vi "Calibrate_Open_All_Freqs-NEW.vi"(8 "error in":errorcluster, 10 "Stop Test":bool, 11 "Calibration Test":bool) -> (0 "error out":errorcluster, 5 "Open Calibration Successful":bool)   [LabVIEW 2020]
uses:
  <vilib>/Utility/error.llb/DialogType.ctl
panel:
  out "message":string=" INSTRUCTIONS:\r\rNormal Use:  When using subVIs that incorporate the error in/error out (or error I/O) structure, place this handler where you want to inform the user of an error, typically at the end of the I/O data path, as the last action of the program.  If the error in error? is ERROR, the handler creates a message describing the error and its source.  If the type of dialog = 1 (default), the message is displayed to the user, who can only acknowedge it.  If the type = 2, the user can acknowledge the message or abort execution; aborting a program with active I/O is not recommended.  If the type = 0, no message is displayed; this is used to process the error programmatically, and the error out cluster elements are wired to individual terminals for that reason.  \r\rOther Use:\n\r\nlocal testing.  To test the error code of a subVI or function that does not have the error I/O structure, you can wire its error code and a source string to the local error code and error source inputs.  If error in error? indicates no error and error code is not equal to 0, the local code and source are substituted for the error in values, and error? is set TRUE (ERROR)."
  out "Test Count":i32
  out "Failed Test Count":i32
  in  "Cal_Delay_Step":u16
  out "serial poll byte":i16
  in  "Test Failed":bool
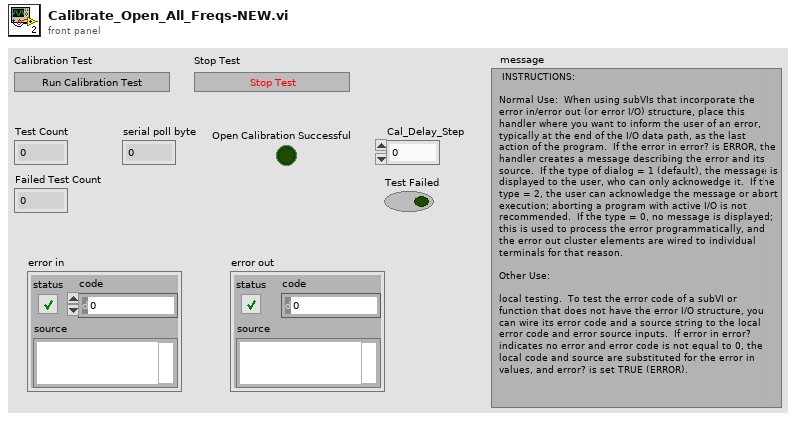
[diagram p1: front panel]
types:
  T1 = typedef "DialogType.ctl" = u16
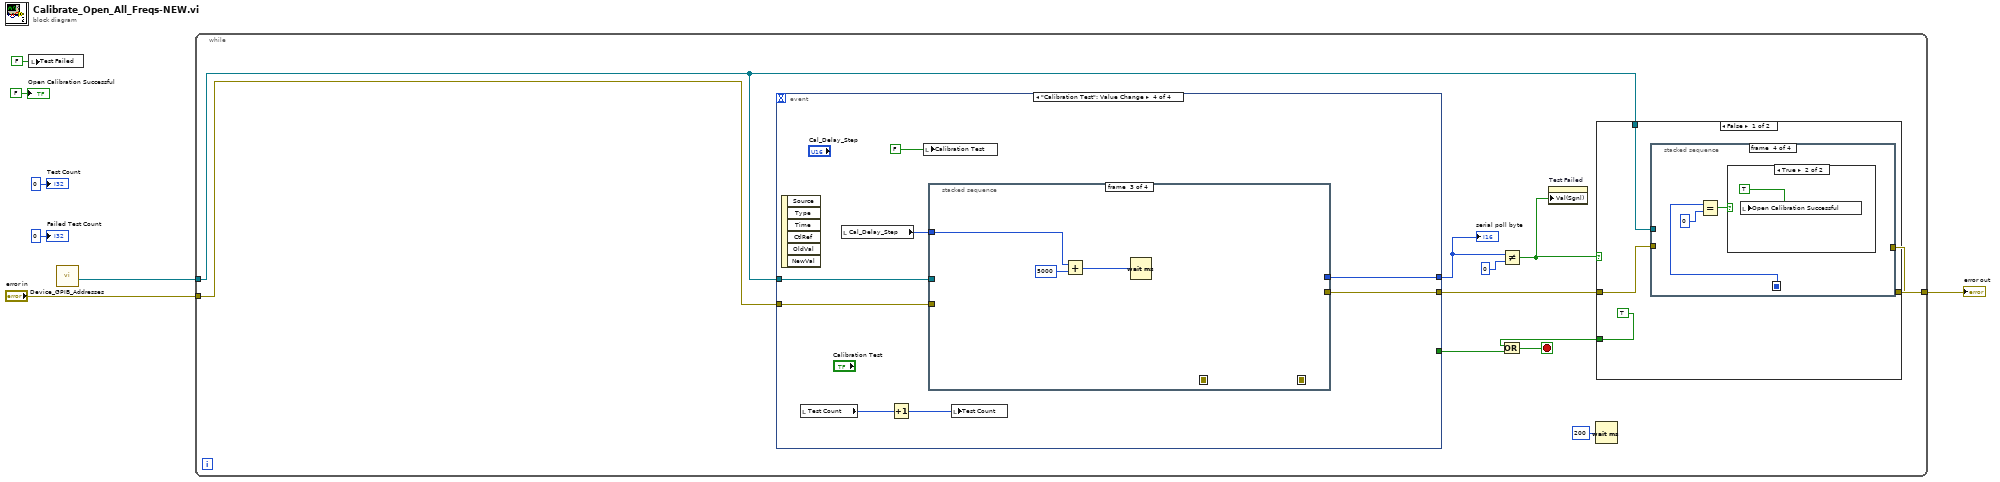
[diagram p0: block diagram]
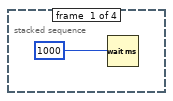
[diagram p2: hidden frame]
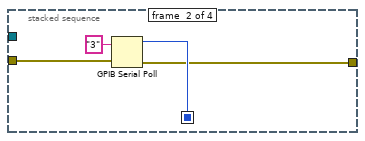
[diagram p3: hidden frame]
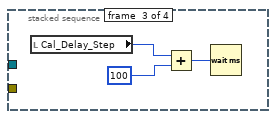
[diagram p4: hidden frame]
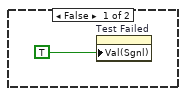
[diagram p5: hidden frame]
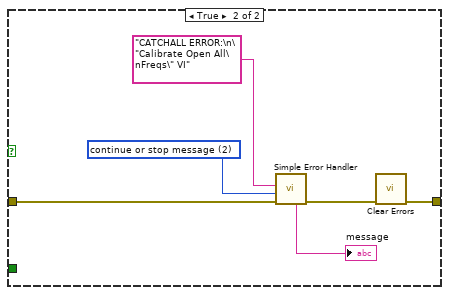
[diagram p6: hidden frame]
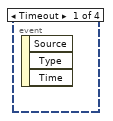
[diagram p7: hidden frame]
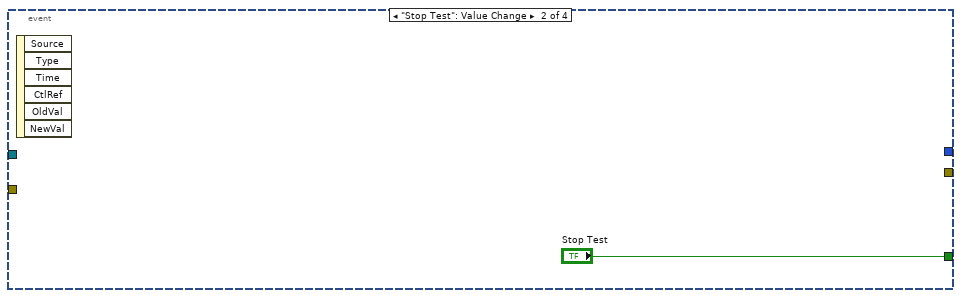
[diagram p8: hidden frame]
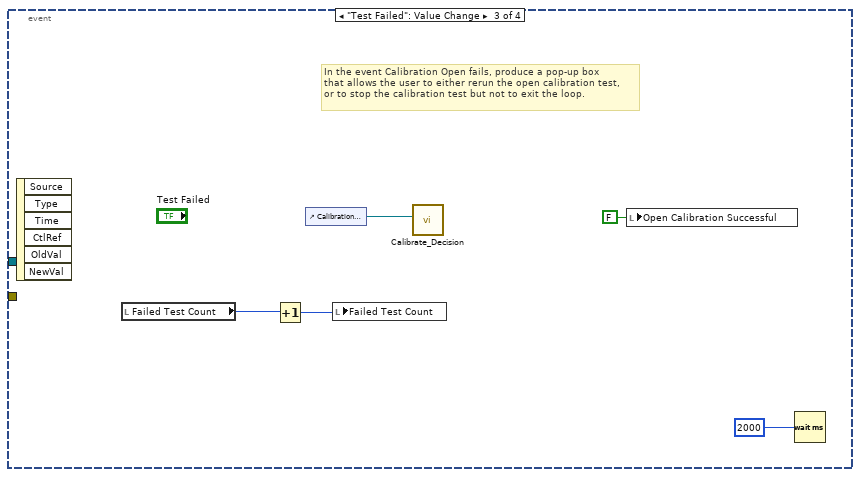
[diagram p9: hidden frame]
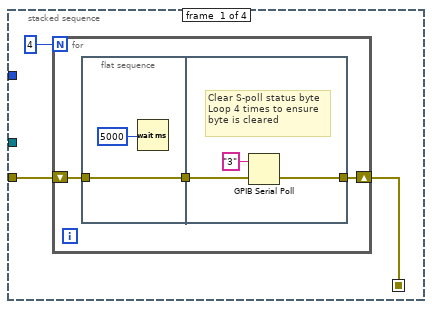
[diagram p10: hidden frame]
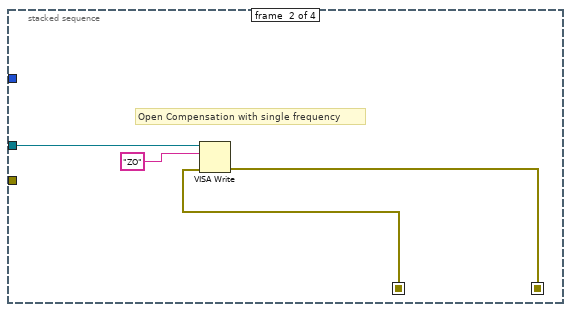
[diagram p11: hidden frame]
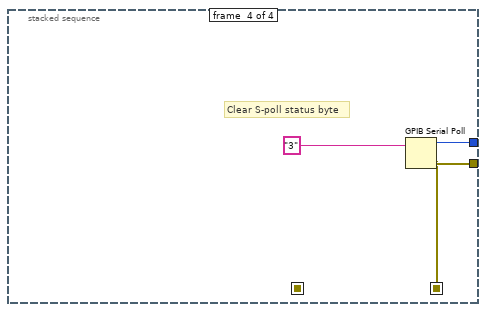
[diagram p12: hidden frame]
diagram:
  n1 = local write "Test Failed"(FALSE ("Test Failed")) -> ()
  n2 = call "Device_GPIB_Addresses.vi"() -> ("HP 4275A Address"=w5:refnum<visa-resource-name>)  [unwired: 9 in, 2 out]
  n3 = while {
    tunnel: w5 -> [w9]
    tunnel: [w17] -> w4
    tunnel: "error in" -> [w8]
    stop <- w13 stop-if-true
    n4 = event shown="[3] \"Calibration Test\": Value Change" {
      selector: _ -> [_ _ _ _]
      dyn-events: _ -> [_ _ _ _]
      timeout: _ -> [_ _ _ _]
      tunnel: [_ "Stop Test" _ _] -> w14
      tunnel: w9 -> [_ _ _ w51]
      tunnel: [_ _ _ w50] -> w18
      tunnel: [_ _ _ w49] -> w15
      tunnel: w8 -> [_ _ _ w48]
      event Timeout {
        n5 = event-data() -> ()  [unwired: 1 in, 3 out]
      }
      event "Stop Test": Value Change {
        n6 = event-data() -> ()  [unwired: 1 in, 6 out]
      }
      event "Test Failed": Value Change {
        # "In the event Calibration Open fails, produce a pop-up box\nthat allows the user to either rerun the open calibration test,\nor to stop the calibration test but not to exit the loop."
        n7 = event-data() -> ()  [unwired: 1 in, 6 out]
        n8 = local read "Failed Test Count"() -> (w45:i32)
        n9 = Increment(x=w45) -> (x+1=w46:i32)
        n10 = control-ref of="Calibration Test"() -> (w47:refnum<vi>)
        n11 = local write "Failed Test Count"(w46) -> ()
        n12 = call "Calibrate_Decision.vi"("reference"=w47) -> ()  [unwired: 11 in]
        n13 = local write "Open Calibration Successful"(FALSE ("Open Calibration Successful")) -> ()
        n14 = Wait (ms)(milliseconds to wait=u32 2000) -> ()  [unwired: 1 out]
      }
      event "Calibration Test": Value Change {
        n15 = event-data() -> ()  [unwired: 1 in, 6 out]
        n16 = local read "Test Count"() -> (w54:i32)
        n17 = local read "Cal_Delay_Step"() -> (w52:u16)
        n18 = Increment(x=w54) -> (x+1=w53:i32)
        n19 = local write "Calibration Test"(FALSE ("Calibration Test")) -> ()
        n20 = stacked-sequence {
          seq-local: [w56 _ _ _] -> [_ w68 _ _]
          seq-local: [_ w67 _ _] -> [_ _ _ w74]
          tunnel: w48 -> [w57 _ _ _]
          tunnel: w52 -> [_ _ w73 _]
          tunnel: [_ _ _ w77] -> w50
          tunnel: [_ _ _ w76] -> w49
          tunnel: w51 -> [_ w70 _ _]
          frame #0 {
            n21 = for {
              N: 4 -> [_]
              shift-right: [w60] -> w56
              shift-left: w57 -> [w61]
              n22 = flat-sequence {
                tunnel: w61 -> [w63]
                tunnel: [w63] -> w59
                tunnel: [w65] -> w60
                tunnel: w59 -> [w66]
                frame #0 {
                  n23 = Wait (ms)(milliseconds to wait=u32 5000) -> ()  [unwired: 1 out]
                }
                frame #1 {
                  # "Clear S-poll status byte\nLoop 4 times to ensure\nbyte is cleared"
                  n24 = GPIB Serial Poll(0:"3" ("address string"), 1:w66) -> (4:w65:errorcluster)  [unwired: 2 out]
                }
              }
            }
          }
          frame #1 {
            # "Open Compensation with single frequency"
            n25 = VISA Write(VISA resource name=w70, write buffer="ZO" ("data"), error in (no error)=w68) -> (error out=w67:errorcluster)  [unwired: 2 out]
          }
          frame #2 {
            n26 = Add(x=w73, y=u16 5000) -> (x+y=w71:u16)
            n27 = Wait (ms)(milliseconds to wait=w71) -> ()  [unwired: 1 out]
          }
          frame #3 {
            # "Clear S-poll status byte"
            n28 = GPIB Serial Poll(0:"3" ("address string"), 1:w74) -> (2:w76:i16, 4:w77:errorcluster)  [unwired: 1 out]
          }
        }
        n29 = local write "Test Count"(w53) -> ()
      }
    }
    "serial poll byte" <- w15
    n30 = Not Equal?(x=w15, y=i16 0) -> (x != y?=w11:bool)
    n31 = property on="Test Failed" class="Bool (strict)"("Val(Sgnl)"=w11) -> ()  [unwired: 2 in, 2 out]
    n32 = Wait (ms)(milliseconds to wait=u32 200) -> ()  [unwired: 1 out]
    n33 = case shown="False" w11 {
      tunnel: w9 -> [w22 _]
      tunnel: w18 -> [w21 w36]
      tunnel: [w20 w37] -> w17
      tunnel: [TRUE _] -> w12
      frame False {
        n34 = stacked-sequence {
          seq-local: [_ w25 _ _] -> [_ _ _ w33]
          tunnel: w21 -> [_ w27 _ _]
          tunnel: [_ w24 _ _] -> w20
          tunnel: w22 -> [_ _ _ _]
          frame #0 {
            n35 = Wait (ms)(milliseconds to wait=u16 1000 ("y")) -> ()  [unwired: 1 out]
          }
          frame #1 {
            n36 = GPIB Serial Poll(0:"3" ("address string"), 1:w27) -> (2:w25:i16, 4:w24:errorcluster)  [unwired: 1 out]
          }
          frame #2 {
            n37 = local read "Cal_Delay_Step"() -> (w28:u16)
            n38 = Add(x=w28, y=u16 100) -> (x+y=w29:u16)
            n39 = Wait (ms)(milliseconds to wait=w29) -> ()  [unwired: 1 out]
          }
          frame #3 {
            n40 = Equal?(x=w33, y=i16 0) -> (x = y?=w31:bool)
            n41 = case shown="True" w31 {
              frame False {
                n42 = property on="Test Failed" class="Bool (strict)"("Val(Sgnl)"=TRUE ("Test Failed")) -> ()  [unwired: 2 in, 2 out]
              }
              frame True {
                n43 = local write "Open Calibration Successful"(TRUE ("Open Calibration Successful")) -> ()
              }
            }
          }
        }
      }
      frame True {
        w39 = T1 2 items=["no dialog", "OK message", "continue or stop message", "OK message + warnings", "continue/stop + warnings"] ("type of dialog (OK msg:1)")
        n44 = call <vilib>:"Simple Error Handler.vi"("error source (\" \")"="CATCHALL ERROR:\n\"Calibrate Open All\nFreqs\" VI" ("error source (\" \")"), "type of dialog (OK msg:1)"=w39, "error in (no error)"=w36) -> ("error out"=w40:errorcluster, "message"=→"message":string)  [unwired: 2 in, 3 out]
        n45 = call <vilib>:"Clear Errors.vi"("error in (no error)"=w40) -> ("error out"=w37:errorcluster)  [unwired: 5 in, 1 out]
      }
    }
    n46 = Or(x=w12, y=w14) -> (x .or. y?=w13:bool)
  }
  "error out" <- w4
  "Failed Test Count" <- 0 ("Failed Test Count")
  "Test Count" <- 0 ("Numeric")
  "Open Calibration Successful" <- FALSE ("Open Calibration Successful")
